vi "SW_Generate_Color_Ramp.vi"(1 "Colors rel. pos.":dbl[](array[numeric]), 2 "Colors array":u32[](array[colorbox])=[16711680, 16773418, 6618880, 9567230, 255]) -> (0 "Colors array":u32[](array[colorbox]))   [LabVIEW 2018, in "Tracker.lvlib"]
uses:
  Tracker.lvlib
panel:
  out "Color array size":i32
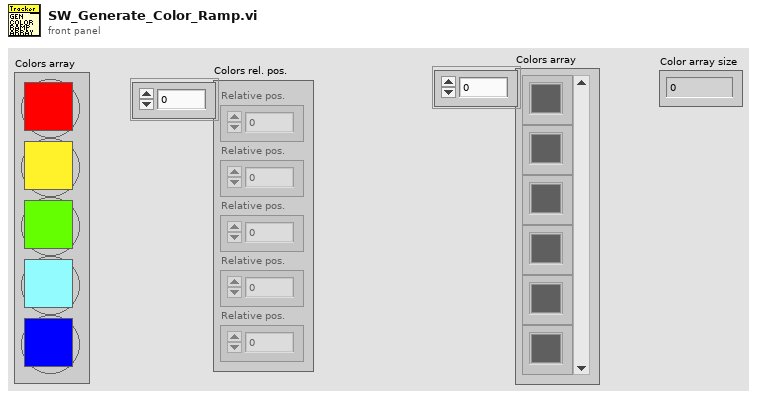
[diagram p1: front panel]
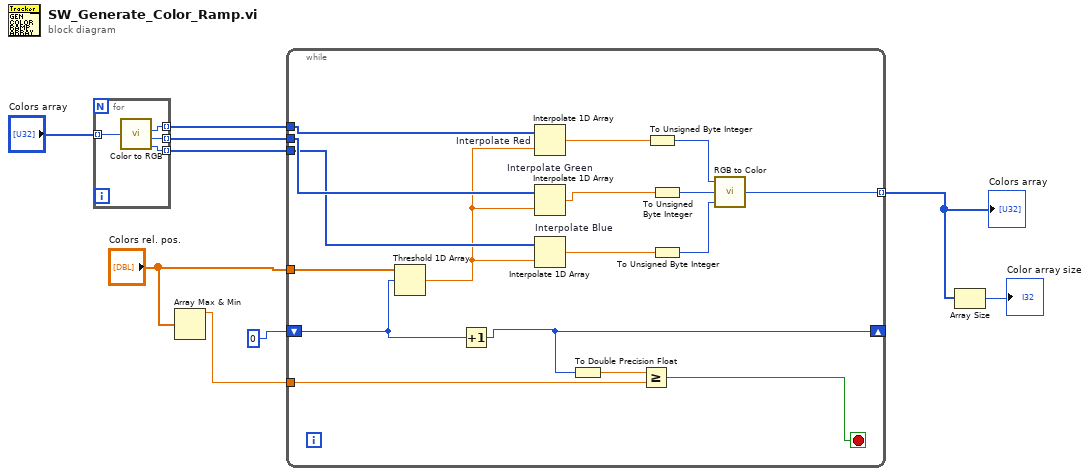
[diagram p0: block diagram]
diagram:
  n1 = for {
    tunnel: [w13] -> w8 mode=indexing
    tunnel: [w12] -> w7 mode=indexing
    tunnel: [w11] -> w6 mode=indexing
    tunnel: "Colors array" -> [w10] mode=indexing
    n2 = call <vilib>:"Color to RGB.vi"("Color"=w10) -> ("R"=w13:u8, "G"=w12:u8, "B"=w11:u8)  [unwired: 1 out]
  }
  n3 = Array Max & Min(array="Colors rel. pos.") -> (max value=w1:dbl)  [unwired: 3 out]
  n4 = while {
    tunnel: "Colors rel. pos." -> [w30]
    tunnel: w8 -> [w29]
    tunnel: w7 -> [w28]
    tunnel: w6 -> [w27]
    tunnel: [w22] -> w4 mode=indexing
    shift-right: [w20] -> _
    shift-left: 0 -> [w21]
    tunnel: w1 -> [w18]
    stop <- w19 stop-if-true
    n5 = Threshold 1D Array(2:w21, 3:w30) -> (0:w26:dbl)  [unwired: 1 in]
    n6 = Increment(x=w21) -> (x+1=w20:i32)
    n7 = Interpolate 1D Array "Interpolate Red"(1:w26, 2:w29) -> (0:w25:dbl)
    n8 = Interpolate 1D Array "Interpolate Green"(1:w26, 2:w28) -> (0:w24:dbl)
    n9 = Interpolate 1D Array "Interpolate Blue"(1:w26, 2:w27) -> (0:w23:dbl)
    n10 = To Double Precision Float(number=w20) -> (double precision float=w14:dbl)
    n11 = Greater Or Equal?(x=w14, y=w18) -> (x >= y?=w19:bool)
    n12 = To Unsigned Byte Integer(number=w25) -> (unsigned 8bit integer=w17:u8)
    n13 = To Unsigned Byte Integer(number=w24) -> (unsigned 8bit integer=w16:u8)
    n14 = To Unsigned Byte Integer(number=w23) -> (unsigned 8bit integer=w15:u8)
    n15 = call <vilib>:"RGB to Color.vi"("B"=w15, "G"=w16, "R"=w17) -> ("Color"=w22:u32)
  }
  "Colors array" <- w4
  n16 = Array Size(array=w4) -> (size(s)=→"Color array size":i32)
